vi "TEST - Close Generic Object Refnum.vi"(8 "error in (no error)":errorcluster) -> (0 "error out":errorcluster, 2 "pass":bool)   [LabVIEW 2009]
uses:
  source/library/Close Generic Object Refnum/Close Generic Object Refnum (Scalar VI).vi
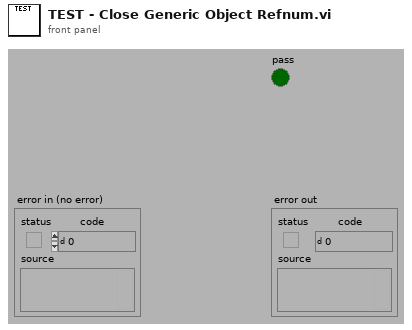
[diagram p1: front panel]
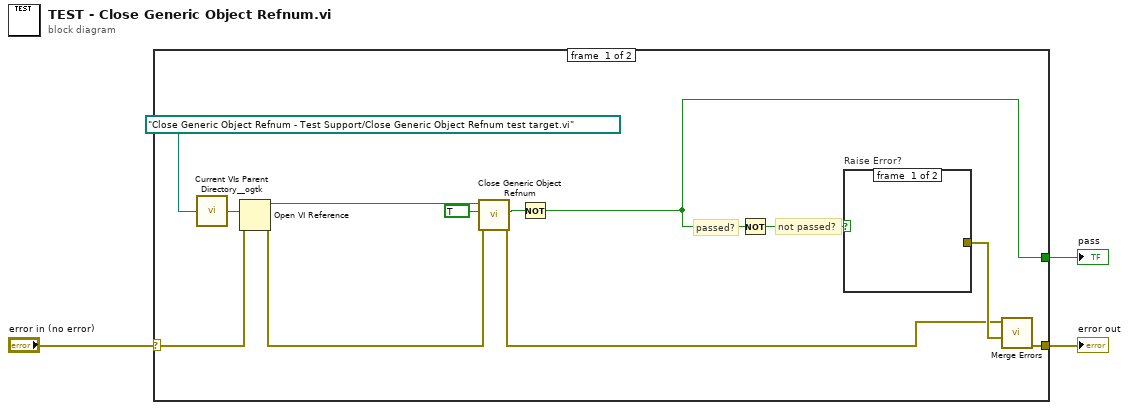
[diagram p0: block diagram]
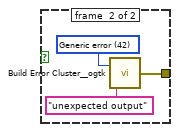
[diagram p2: hidden frame]
diagram:
  n1 = case shown="No Error" "error in (no error)" {
    selector: "error in (no error)" -> [w12 w19]
    tunnel: [w4 _] -> w3
    tunnel: [w15 w19] -> w1
    frame #0 {
      # "not passed?"
      # "passed?"
      n2 = call <userlib>:"Current VIs Parent Directory__ogtk.vi"("Relative path (.)"=path "Close Generic Object Refnum - Test Support/Close Generic Object Refnum test target.vi") -> ("Parent Directory (+ Relative)"=w11:path)  [unwired: 4 in]
      n3 = Open VI Reference(vi path=w11, error in (no error)=w12) -> (vi reference=w8:refnum<vi>, error out=w9:errorcluster)  [unwired: 4 in]
      n4 = call-poly "Close Generic Object Refnum.vi"("error in (no error)"=w9, "wait on unloaded? (FALSE)"=TRUE, "VI Refnum"=w8) -> ("error out"=w6:errorcluster, "timed out?"=w5:bool)  [unwired: 7 in]
      n5 = Not(x=w5) -> (.not. x?=w4:bool)
      n6 = Not(x=w4) -> (.not. x?=w14:bool)
      n7 = case "Raise Error?" shown="True" w14 {
        tunnel: [_ w16] -> w10
        frame #0 {
        }
        frame #1 {
          w17 = 42 items=["No error", "Argument error", "Memory is full", "Out of zone", "End of file", "File already open", "Generic file I/O error", "File not found", "File permission error", "Disk is full", "Duplicate path", "Too many files open", "System feature not enabled", "Resource file not found", "Cannot add resource", "Resource not found", "Image not found", "Image memory error", "Pen does not exist", "Config type invalid", "Config token not found", "Config parse error", "Config memory error", "Bad external code format", "Bad external code offset", "External code not present", "Null window", "Destroy window error", "Null menu", "Print aborted", "Bad print record", "Print driver error", "Windows error during printing", "Memory error during printing", "Print dialog error", "Generic print error", "Invalid device refnum", "Device not found", "Device parameter error", "Device unit error", "Cannot open device", "Device call aborted", "Generic error", "Cancelled by user", "Object ID too low", "Object ID too high", "Object not in heap", "Unknown heap", "Unknown object (invalid DefProc)", "Unknown object (DefProc not in table)", "Message out of range", "Invalid (null) method", "Unknown message", "Manager call not supported", "Bad address", "Network operation in progress", "Network operation timed out", "Connection is busy", "Network attribute not supported", "Network error", "Address in use", "System out of memory", "Connection aborted", "Connection refused", "Not connected", "Already connected", "Connection closed", "Initialization error (interapplication manager)", "Bad occurrence", "Wait on unbound occurrence handler", "Occurrence queue overflow", "Datalog type conflict", "Unused", "Unrecognized type (interapplication manager)", "Memory corrupt", "Failed to make temporary DLL", "Old CIN version", "Drag socket not found", "Failed to load drop-object", "Failed to register OLE object", "Failed to release OLE object", "Format specifier type mismatch", "Unknown format specifier", "Too few format specifiers", "Too many format specifiers", "Scan failed", "Newer CIN version", "Error converting to variant", "Runtime menu error", "Password tampered", "Variant attribute not found", "Incompatible variant data type", "Event data is not available", "Event Store is not present", "Occurrence is not found", "Event Queue is not created", "Event info is not available", "Refnum passed is NULL", "Error retrieving Class GUID", "Error retrieving CoClass GUID", "Error retrieving TypeLib GUID.", "Bad built application magic bytes.", "Specific driver is different from the specific driver associated with the Logical Name.", "There is no session opened to the class driver.", "Max Error", "MAX - Error with config objects", "MAX - Error loading configuration", "MAX - Group not supported"]
          n8 = call <userlib>:"Build Error Cluster__ogtk.vi"("String to Prepend to source (\"\")"="unexpected output" ("String to Prepend to source (\"\")"), "code"=w17) -> ("error out"=w16:errorcluster)
        }
      }
      n9 = call <vilib>:"Merge Errors.vi"("error in 3 (no error)"=w10, "error in 1 (no error)"=w6) -> ("error out"=w15:errorcluster)  [unwired: 5 in]
    }
    frame #1 {
    }
  }
  "pass" <- w3
  "error out" <- w1
